vi "Write.vi"(8 "error in (no error)":errorcluster, 10 "String":string, 11 "Boolean in":refnum<class "Blackboard_String.lvclass">) -> (0 "error out":errorcluster, 3 "Boolean out":refnum<class "Blackboard_String.lvclass">)   [LabVIEW 2021, in "Blackboard_String.lvclass"]
doc: "Abstract Data Classes 2.1.1.12\nTim Streeter - TSA\nCopyright (c) 2024, TSA"
uses:
  Blackboard_String.lvclass
  Blackboard_String.lvclass/Blackboard_String.ctl
  Blackboard.lvclass
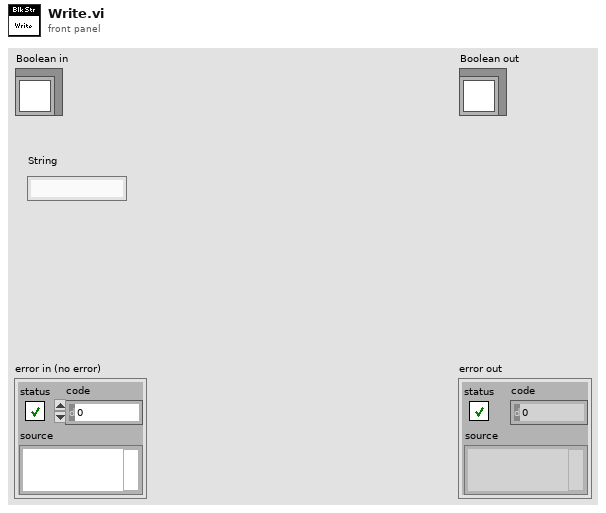
[diagram p1: front panel]
types:
  T1 = typedef "Blackboard.lvclass/Data DVR Type.ctl" = cluster{"Tags":T2, "Status":refnum<data-value>, "Boolean":refnum<data-value>, "String":refnum<data-value>, "DBL":refnum<data-value>, "SGL":refnum<data-value>, "EXT":refnum<data-value>, "U8":refnum<data-value>, "U16":refnum<data-value>, "U32":refnum<data-value>, "U64":refnum<data-value>, "I8":refnum<data-value>, "I16":refnum<data-value>, "I32":refnum<data-value>, "I64":refnum<data-value>, "CDBL":refnum<data-value>, "CSGL":refnum<data-value>, "CEXT":refnum<data-value>, "Time":refnum<data-value>, "Variant":refnum<data-value>, "Waveform":refnum<data-value>}
  T2 = typedef "Blackboard.lvclass/Tags Map Type.ctl" = map{string, cluster{"Data Index":i32, "Status Index":i32}}
  T3 = typedef "Blackboard.lvclass/Group Map Type.ctl" = map{string, i32}
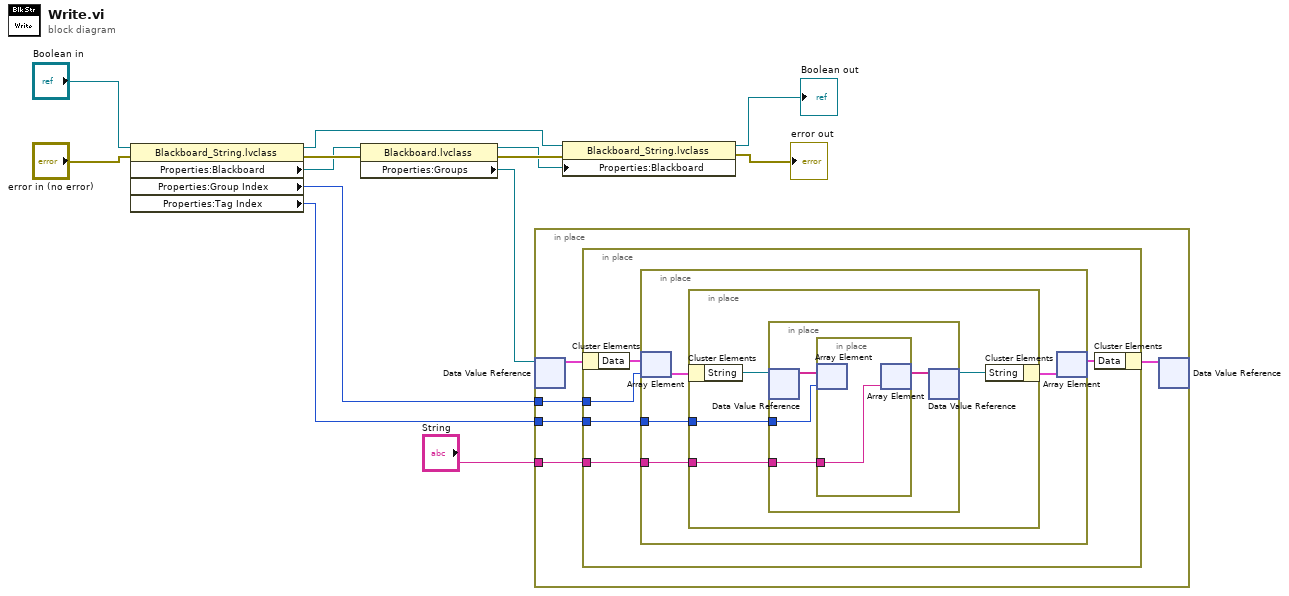
[diagram p0: block diagram]
diagram:
  n1 = property class="Blackboard_String.lvclass"(reference="Boolean in", error in="error in (no error)") -> (reference out=w7:refnum<class "Blackboard_String.lvclass">, error out=w13:errorcluster, "Properties:Blackboard"=w8:refnum<class "Blackboard.lvclass">, "Properties:Group Index"=w12:i32, "Properties:Tag Index"=w9:i32)
  n2 = property class="Blackboard.lvclass"(reference=w8, error in=w13) -> (reference out=w10:refnum<class "Blackboard.lvclass">, error out=w11:errorcluster, "Properties:Groups"=w1:refnum<data-value>)
  n3 = in-place {
    in-place-border: w12 -> [w18]
    in-place-border: w9 -> [w17]
    in-place-border: "String" -> [w16]
    n4 = in-place-dvr #1(w1) -> (w15:cluster{"Data":T1[], "Map":T3, "Status":u32[]})  [unwired: 1 out]
    n5 = in-place {
      in-place-border: w18 -> [w23]
      in-place-border: w17 -> [w22]
      in-place-border: w16 -> [w21]
      n6 = in-place-cluster #2(w15) -> ("Data"=w20:T1[])
      n7 = in-place {
        in-place-border: w22 -> [w26]
        in-place-border: w21 -> [w25]
        n8 = in-place-array #3(w20, w23) -> (w27:T1)
        n9 = in-place {
          in-place-border: w26 -> [w29]
          in-place-border: w25 -> [w28]
          n10 = in-place-cluster #4(w27) -> ("String"=w31:refnum<data-value>)
          n11 = in-place {
            in-place-border: w29 -> [w33]
            in-place-border: w28 -> [w32]
            n12 = in-place-dvr #5(w31) -> (w35:string[])  [unwired: 1 out]
            n13 = in-place {
              in-place-border: w32 -> [w36]
              n14 = in-place-array #6(w35, w33) -> ()  [unwired: 1 out]
              n15 = in-place-array #6(w36) -> (w34:string[])  [unwired: 1 out]
            }
            n16 = in-place-dvr #5(w34) -> (w30:refnum<data-value>)  [unwired: 1 out]
          }
          n17 = in-place-cluster #4("String"=w30) -> (w24:T1)
        }
        n18 = in-place-array #3(w24) -> (w19:T1[])  [unwired: 1 out]
      }
      n19 = in-place-cluster #2("Data"=w19) -> (w14:cluster{"Data":T1[], "Map":T3, "Status":u32[]})
    }
    n20 = in-place-dvr #1(w14) -> ()  [unwired: 2 out]
  }
  n21 = property class="Blackboard_String.lvclass"(reference=w7, error in=w11, "Properties:Blackboard"=w10) -> (reference out=→"Boolean out":refnum<class "Blackboard_String.lvclass">, error out=→"error out":errorcluster)
